vi "Initialize.vi"(8 "error in":errorcluster, 9 "PPLs Folder Path":path, 10 "INI File Path":path, 11 "Device":string) -> (0 "error out":errorcluster, 3 "Camera out":refnum<class "Camera.lvclass">)   [LabVIEW 2018, in "Camera.lvlib" / "Camera.lvclass"]
uses:
  Camera.lvclass
  Camera.lvclass/Camera.ctl
  PPLs/Configuration/Configuration.lvlibp/Configuration.lvclass
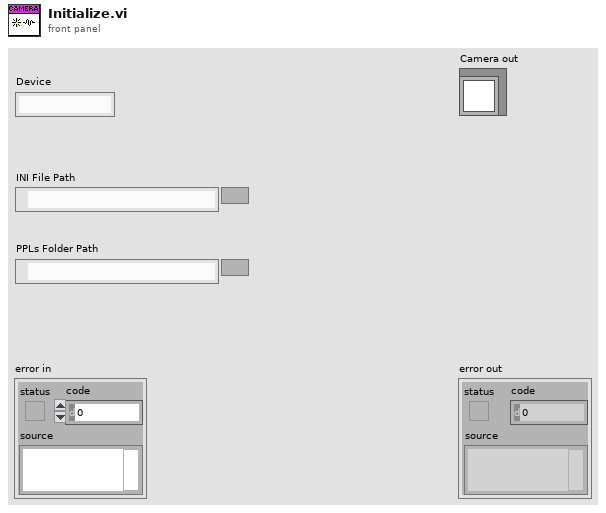
[diagram p1: front panel]
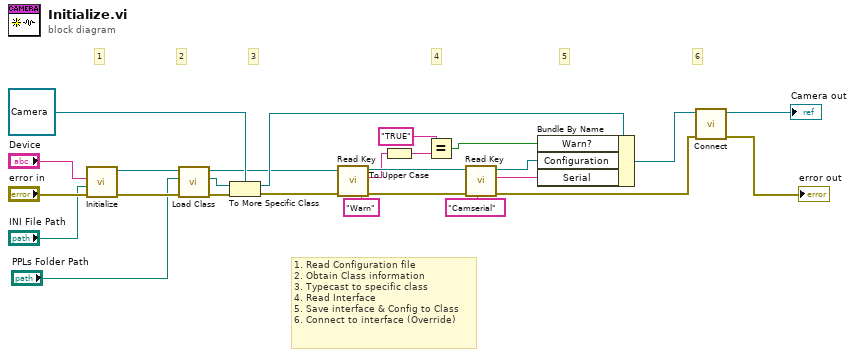
[diagram p0: block diagram]
diagram:
  # "6"
  # "5"
  # "4"
  # "3"
  # "2"
  # "1"
  # "1. Read Configuration file\n2. Obtain Class information\n3. Typecast to specific class\n4. Read Interface\n5. Save interface & Config to Class\n6. Connect to interface (Override)"
  n1 = call "Initialize.vi"("error in"="error in", "INI File Path"="INI File Path", "Device"="Device") -> ("error out"=w21:errorcluster, "Configuration out"=w22:refnum<class "Configuration.lvclass">)  [unwired: 7 in]
  n2 = call "Load Class.vi"("error in"=w21, "PPLs Folder Path"="PPLs Folder Path", "Configuration in"=w22) -> ("error out"=w20:errorcluster, "Class out"=w19:refnum<class>, "Configuration out"=w8:refnum<class "Configuration.lvclass">)  [unwired: 6 in]
  n3 = To More Specific Class(target class=refnum<class "Camera.lvclass"> refnum ("Camera in"), reference=w19, error in=w20) -> (specific class reference=w17:refnum<class "Camera.lvclass">, error out=w11:errorcluster)
  n4 = call "Read Key.vi"("Key:"="Warn", "error in"=w11, "Configuration in"=w8) -> ("error out"=w10:errorcluster, "Value"=w6:string, "Configuration out"=w9:refnum<class "Configuration.lvclass">)  [unwired: 6 in]
  n5 = To Upper Case(1:w6) -> (0:w5:string)
  n6 = Equal?(x="TRUE", y=w5) -> (x = y?=w4:bool)
  n7 = call "Read Key.vi"("Key:"="Camserial", "error in"=w10, "Configuration in"=w9) -> ("error out"=w13:errorcluster, "Value"=w16:string, "Configuration out"=w15:refnum<class "Configuration.lvclass">)  [unwired: 6 in]
  n8 = Bundle By Name(cluster=w17, "Warn?"=w4, "Configuration"=w15, "Serial"=w16) -> (w14:refnum<class "Camera.lvclass">)
  n9 = call-dynamic "Connect.vi"("error in (no error)"=w13, "Camera in"=w14) -> ("error out"=→"error out":errorcluster, "Camera out"=→"Camera out":refnum<class "Camera.lvclass">)  [unwired: 8 in]
